vi "Gss.vi"() -> ()   [LabVIEW 2016]
panel:
  out "GssDagger":dbl[][](array[numeric])
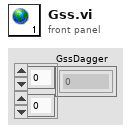
[diagram p1: front panel]
diagram:
